vi "Encode Section and Key Names__ogtk.vi"(7 "use legacy encoding scheme? (FALSE)":bool, 10 "string":string) -> (2 "encoded string":string)   [LabVIEW 2016]
doc: "Encodes and decodes section and key names.\n\nEscapes the following:\n\n \\ (escape code special character escaped as \\\\)\n \\00-\\1F (non-printable chars)\n \"[\", \"]\", and \"=\" (INI syntax elements)\n \\FE (\"þ\") and \\FF (\"ÿ\") (legacy encoding)\n\nLegacy encoding encodes brackets, \"[\" and \"]\", as special characters \"þ\" and \"ÿ\"."
panel:
  # "Encode Section and Key Names.vi\n\nEncodes and decodes section and key names.\n\nPlease visit http://www.OpenG.org to learn about the\nOpen Source LabVIEW software movement.\n\nNOTICE -- YOU MUST LEAVE THIS NOTICE IN PLACE.  PER THE TERMS OF THE LICENSE BELOW, YOU MAY SUBLICENSE THIS SOFTWARE \nIN ANY WAY THAT DOES NOT CONFLICT WITH THIS LICENSE.\n\n### BSD License (http://www.opensource.org/licenses/bsd-license.php) Begin ###\n \nCopyright (c) 2004, Heiko Fettig <Heiko.Fettig@gmx.net>\nCopyright (c) 2006, Jim Kring <jim@jimkring.com>\n\nAll rights reserved.\n\nRedistribution and use in source and binary forms, with or without modification, are permitted provided that the following conditions are met:\n\n    * Redistributions of source code must retain the above copyright notice, this list of conditions and the following disclaimer.\n    * Redistributions in binary form must reproduce the above copyright notice, this list of conditions and the following disclaimer in the \n       documentation and/or other materials provided with the distribution.\n    * Neither the name of SciWare, James Kring, Inc., nor the names of its contributors may be used to endorse or promote products derived \n       from this software without specific prior written permission.\n\nTHIS SOFTWARE IS PROVIDED BY THE COPYRIGHT HOLDERS AND CONTRIBUTORS \"AS IS\" AND ANY EXPRESS OR IMPLIED WARRANTIES, \nINCLUDING, BUT NOT LIMITED TO, THE IMPLIED WARRANTIES OF MERCHANTABILITY AND FITNESS FOR A PARTICULAR PURPOSE ARE \nDISCLAIMED. IN NO EVENT SHALL THE COPYRIGHT OWNER OR CONTRIBUTORS BE LIABLE FOR ANY DIRECT, INDIRECT, INCIDENTAL,\n SPECIAL, EXEMPLARY, OR CONSEQUENTIAL DAMAGES (INCLUDING, BUT NOT LIMITED TO, PROCUREMENT OF SUBSTITUTE GOODS OR \nSERVICES; LOSS OF USE, DATA, OR PROFITS; OR BUSINESS INTERRUPTION) HOWEVER CAUSED AND ON ANY THEORY OF LIABILITY, \nWHETHER IN CONTRACT, STRICT LIABILITY, OR TORT (INCLUDING NEGLIGENCE OR OTHERWISE) ARISING IN ANY WAY OUT OF THE USE \nOF THIS SOFTWARE, EVEN IF ADVISED OF THE POSSIBILITY OF SUCH DAMAGE.\n\n### BSD License End ###"
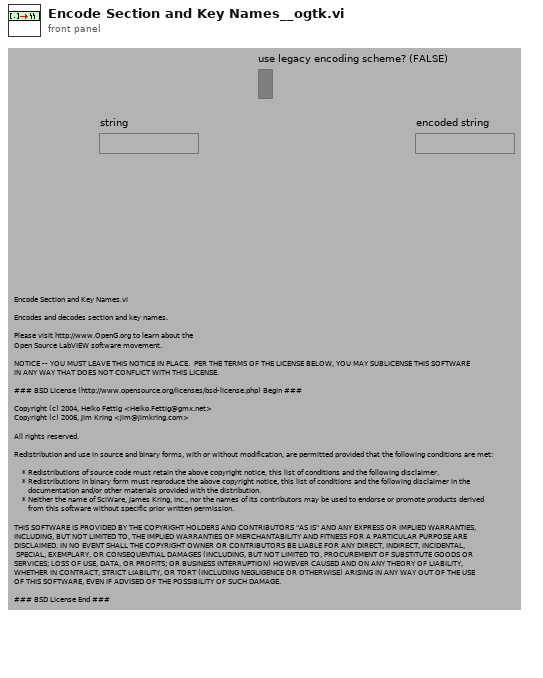
[diagram p1: front panel]
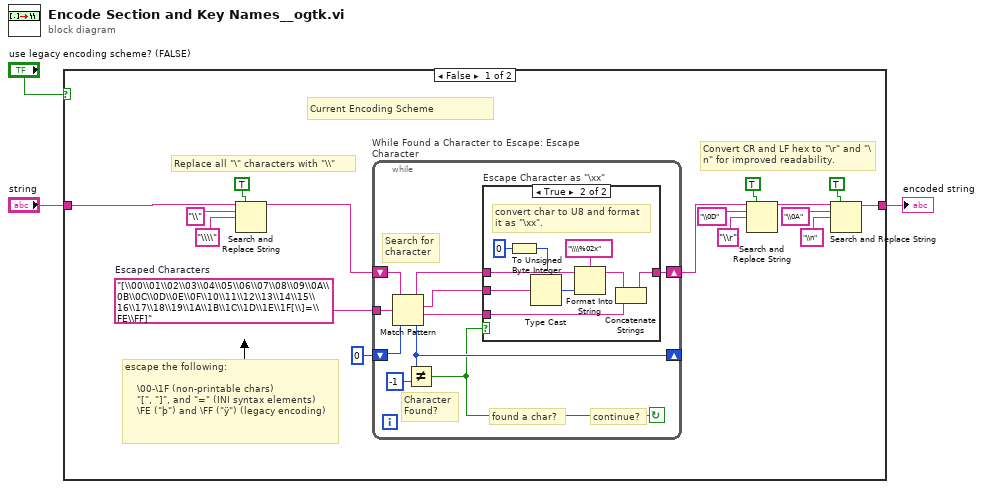
[diagram p0: block diagram]
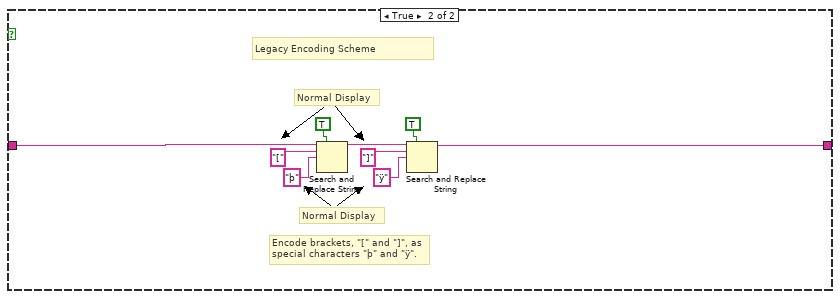
[diagram p3: hidden frame]
diagram:
  n1 = case shown="False" "use legacy encoding scheme? (FALSE)" {
    tunnel: [w4 w41] -> w3
    tunnel: "string" -> [w13 w40]
    frame False {
      w19 = "[\\00\\01\\02\\03\\04\\05\\06\\07\\08\\09\\0A\\0B\\0C\\0D\\0E\\0F\\10\\11\\12\\13\\14\\15\\16\\17\\18\\19\\1A\\1B\\1C\\1D\\1E\\1F[\\]=\\FE\\FF]"  # Escaped Characters
      # "Convert CR and LF hex to \"\\r\" and \"\\n\" for improved readability."
      # "Current Encoding Scheme"
      # "Replace all \"\\\" characters with \"\\\\\""
      # "escape the following:\n\n    \\00-\\1F (non-printable chars)\n    \"[\", \"]\", and \"=\" (INI syntax elements)\n    \\FE (\"þ\") and \\FF (\"ÿ\") (legacy encoding)"
      n2 = Search and Replace String(replace all?=TRUE ("replace all? (F)"), input string=w13, search string="\\", replace string="\\\\" ("replace string (\"\")")) -> (result string=w14:string)  [unwired: 4 in, 3 out]
      n3 = while "While Found a Character to Escape: Escape Character" {
        tunnel: w19 -> [w29]
        shift-right: [w21] -> w9
        shift-left: w14 -> [w24]
        shift-right: [w28] -> _
        shift-left: 0 ("offset past match") -> [w20]
        stop <- w26 continue-if-true
        # "continue?"
        # "Search for character"
        # "found a char?"
        # "Character Found?"
        n4 = Match Pattern(string=w24, regular expression=w29, offset (0)=w20) -> (before substring=w23:string, match substring=w25:string, after substring=w22:string, offset past match=w28:i32)
        n5 = Not Equal?(x=w28, y=-1) -> (x != y?=w26:bool)
        n6 = case "Escape Character as \"\\xx\"" shown="True" w26 {
          tunnel: w25 -> [_ w39]
          tunnel: w23 -> [w30 w35]
          tunnel: w22 -> [_ w33]
          tunnel: [w30 w31] -> w21
          frame False {
          }
          frame True {
            # "convert char to U8 and format it as \"\\xx\"."
            n7 = To Unsigned Byte Integer(number=u8 0) -> (unsigned 8bit integer=w32:u8)
            n8 = Type Cast(type=w32, x=w39) -> (*(type *) &x=w37:u8)
            n9 = Format Into String(format string="\\\\%02x", initial string=w35, w37) -> (resulting string=w34:string)  [unwired: 1 in, 1 out]
            n10 = Concatenate Strings(w34, w33) -> (w31:string)
          }
        }
      }
      n11 = Search and Replace String(replace all?=TRUE ("replace all? (F)"), input string=w9, search string="\\0D", replace string="\\r" ("replace string (\"\")")) -> (result string=w8:string)  [unwired: 4 in, 3 out]
      n12 = Search and Replace String(replace all?=TRUE ("replace all? (F)"), input string=w8, search string="\\0A", replace string="\\n" ("replace string (\"\")")) -> (result string=w4:string)  [unwired: 4 in, 3 out]
    }
    frame True {
      # "Legacy Encoding Scheme"
      # "Normal Display"
      # "Encode brackets, \"[\" and \"]\", as special characters \"þ\" and \"ÿ\"."
      # "Normal Display"
      n13 = Search and Replace String(replace all?=TRUE ("replace all? (F)"), input string=w40, search string="[", replace string="þ" ("replace string (\"\")")) -> (result string=w48:string)  [unwired: 4 in, 3 out]
      n14 = Search and Replace String(replace all?=TRUE ("replace all? (F)"), input string=w48, search string="]", replace string="ÿ" ("replace string (\"\")")) -> (result string=w41:string)  [unwired: 4 in, 3 out]
    }
  }
  "encoded string" <- w3
